vi "Delete Bucket.vi"(8 "error in (no error)":errorcluster, 9 "Bucket":string) -> (0 "error out":errorcluster)   [LabVIEW 2011, in "LV Interface for Amazon S3.lvlib"]
doc: "This operation <B>deletes the specified bucket</B>. <B>NOTE: All objects</B> (including all object versions and Delete Markers) in the bucket <B>must be deleted before</B> the bucket itself can be deleted!"
uses:
  LV Interface for Amazon S3.lvlib
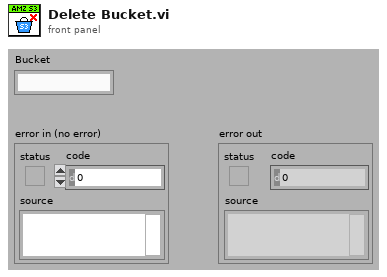
[diagram p1: front panel]
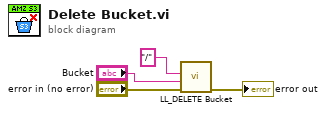
[diagram p0: block diagram]
diagram:
  n1 = call "LL_DELETE Bucket.vi"("error in (no error)"="error in (no error)", "Bucket"="Bucket", "Path and query string"="/") -> ("error out"=→"error out":errorcluster)  [unwired: 7 in, 1 out]
